vi "save_couping.vi"(0 "Apeak":dbl[](array[numeric]), 1 "Apeakpos":dbl[](array[numeric]), 2 "Apeaknext":dbl[](array[numeric]), 3 "Anextpos":dbl[](array[numeric]), 4 "Bpeak":dbl[](array[numeric]), 5 "Bpeakpos":dbl[](array[numeric]), 6 "PATH":string, 7 "Bpeaknext":dbl[](array[numeric]), 8 "Tabsize":dbl, 9 "Bnextpos":dbl[](array[numeric]), 10 "FreqTab":dbl[](array[numeric]), 11 "RApeak":dbl[](array[numeric]), 12 "MODE":dbl, 13 "RApos":dbl[](array[numeric]), 18 "RBpos":dbl[](array[numeric]), 19 "RBpeak":dbl[](array[numeric])) -> ()   [LabVIEW 2015]
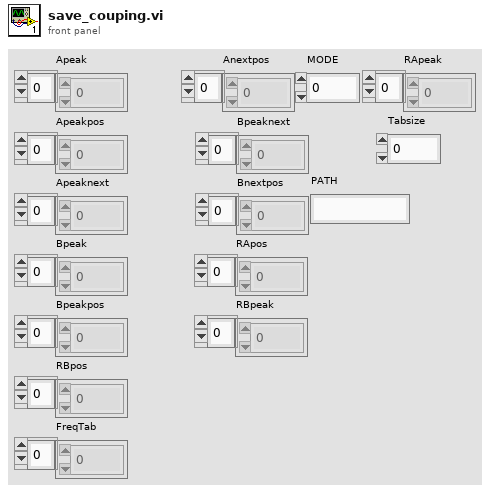
[diagram p1: front panel]
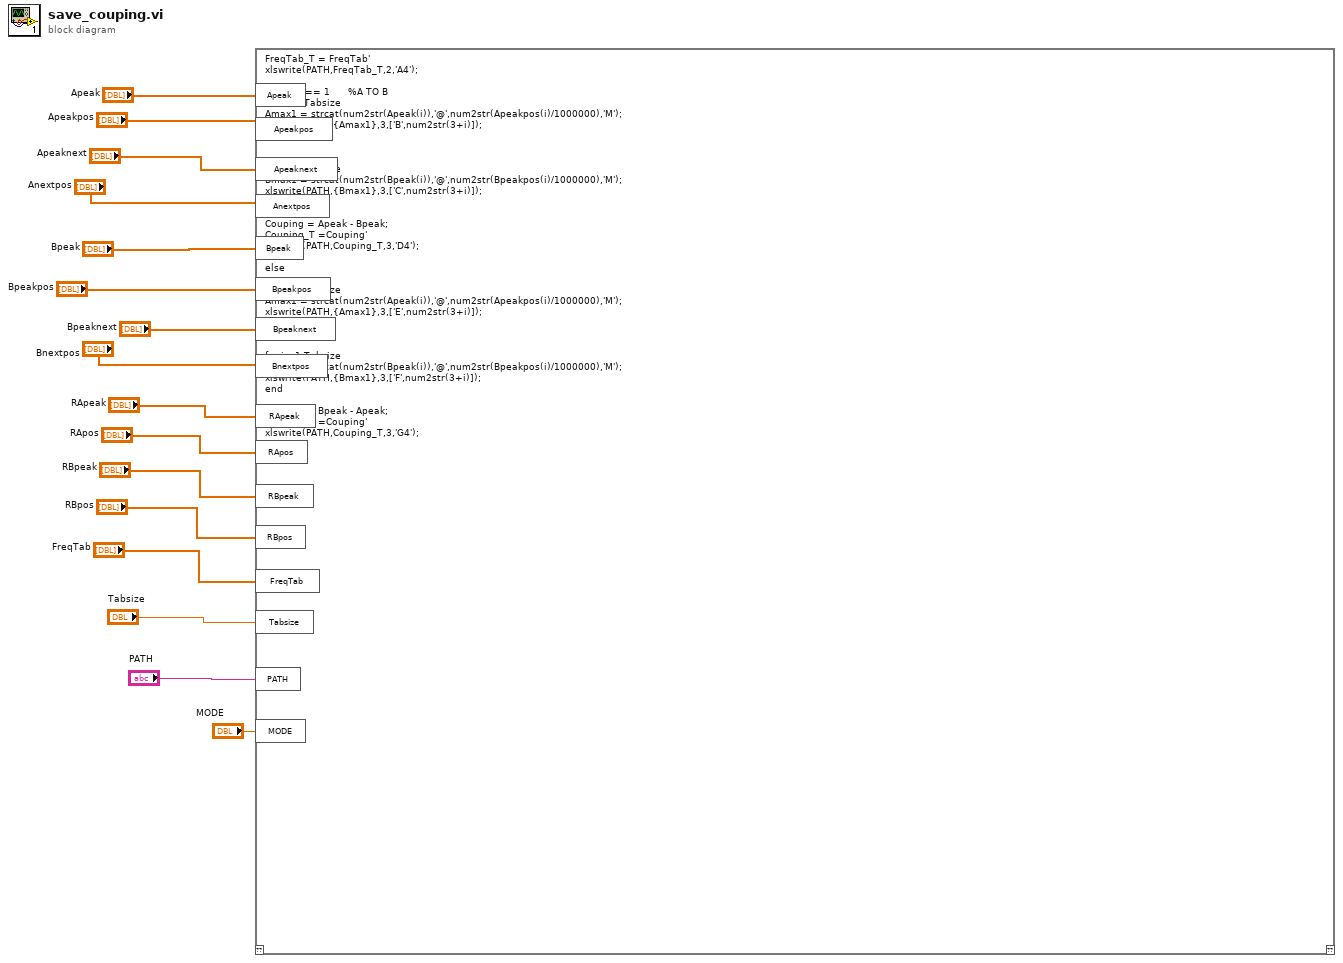
[diagram p0: block diagram]
diagram:
  n1 = script code="FreqTab_T = FreqTab'\nxlswrite(PATH,FreqTab_T,2,'A4');\n\nif MODE == 1      %A TO B\nfor i= 1:Tabsize\nAmax1 = strcat(num2str(Apeak(i)),'@',num2str(Apeakpos(i)/1000000),'M');\nxlswrite(PATH,{Amax1},3,['B',num2str(3+i)]);\nend\n\n\nfor i= 1:Tabsize\nBmax1 = strcat(num2str(Bpeak(i)),'@',num2str(Bpeakpos(i)/1000000),'M');\nxlswrite(PATH,{Bmax1},3,['C',num2str(3+i)]);\nend\n\nCouping = Apeak - Bpeak;\nCouping_T =Couping'\nxlswrite(PATH,Couping_T,3,'D4');\n\nelse\n\nfor i= 1:Tabsize\nAmax1 = strcat(num2str(Apeak(i)),'@',num2str(Apeakpos(i)/1000000),'M');\nxlswrite(PATH,{Amax1},3,['E',num2str(3+i)]);\nend\n\n\nfor i= 1:Tabsize\nBmax1 = strcat(num2str(Bpeak(i)),'@',num2str(Bpeakpos(i)/1000000),'M');\nxlswrite(PATH,{Bmax1},3,['F',num2str(3+i)]);\nend\n\nCouping = Bpeak - Apeak;\nCouping_T =Couping'\nxlswrite(PATH,Couping_T,3,'G4');\n\nend"("Apeak"="Apeak", "Apeakpos"="Apeakpos", "Apeaknext"="Apeaknext", "Anextpos"="Anextpos", "Bpeak"="Bpeak", "Bpeakpos"="Bpeakpos", "Bpeaknext"="Bpeaknext", "Bnextpos"="Bnextpos", "RApeak"="RApeak", "RApos"="RApos", "RBpeak"="RBpeak", "RBpos"="RBpos", "FreqTab"="FreqTab", "Tabsize"="Tabsize", "PATH"="PATH", "MODE"="MODE") -> ()  [unwired: 1 in, 1 out]
